vi "ipg_float.vi"(1 "String":string) -> (0 "Float":sgl)   [LabVIEW 2023, in "Laser_com_2022.lvlib"]
uses:
  Laser_com_2022.lvlib
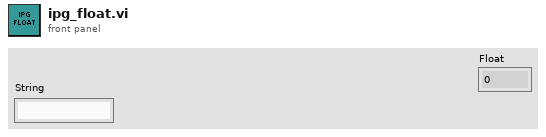
[diagram p1: front panel]
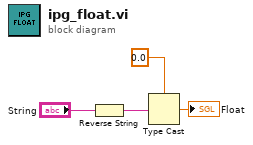
[diagram p0: block diagram]
diagram:
  n1 = Reverse String(1:"String") -> (0:w3:string)
  n2 = Type Cast(type=sgl 0.0, x=w3) -> (*(type *) &x=→"Float":sgl)
